vi "PV ActiveLine - FullScaleRange.vi"   [LabVIEW 2013, in "PV ActiveLine.lvlib"]
uses:
  C:/Program Files (x86)/National Instruments/LabVIEW 2013/PV ActiveLine/PV ActiveLine.lvlib
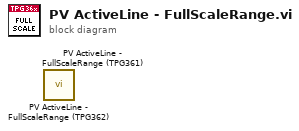
[diagram p0: block diagram]
diagram:
  n1 = call "PV ActiveLine - FullScaleRange (TPG362).vi"() -> ()  [unwired: 8 in, 4 out]
  n2 = call "PV ActiveLine - FullScaleRange (TPG361).vi"() -> ()  [unwired: 9 in, 3 out]
